vi "New QDList.vi"(8 "error in (no error)":errorcluster, 11 "QDDialogList in":refnum<class "QDDialogList.lvclass">) -> (0 "error out":errorcluster, 3 "QDDialogList out":refnum<class "QDDialogList.lvclass">)   [LabVIEW 2015, in "QDDialogList.lvclass"]
uses:
  QDDialogList.lvclass
  QDDialogList.lvclass/QDDialogList.ctl
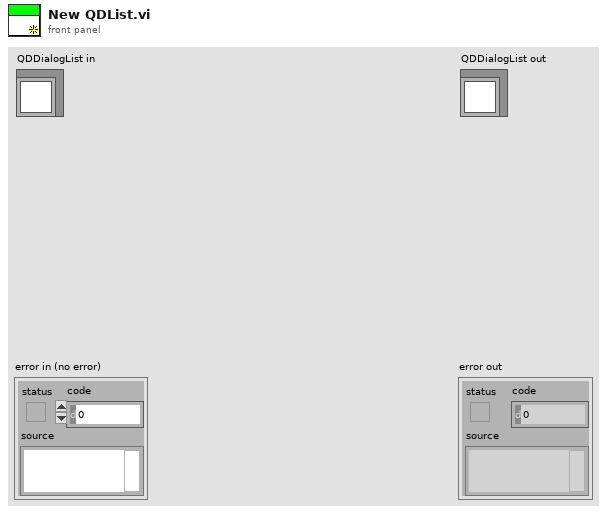
[diagram p1: front panel]
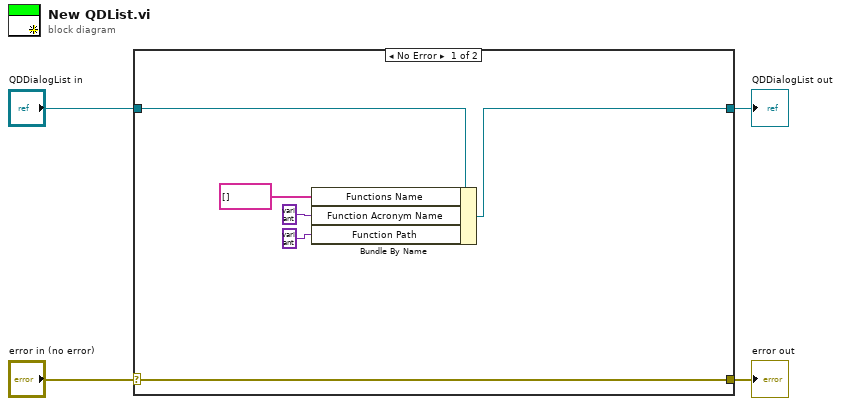
[diagram p0: block diagram]
diagram:
  n1 = case shown="No Error" "error in (no error)" {
    selector: "error in (no error)" -> [w10 w12]
    tunnel: [w10 w12] -> w3
    tunnel: [w5 w11] -> w1
    tunnel: "QDDialogList in" -> [w9 w11]
    frame No Error {
      n2 = Bundle By Name(cluster=w9, "Functions Name"=string[] [], "Function Acronym Name"=variant, "Function Path"=variant) -> (w5:refnum<class "QDDialogList.lvclass">)
    }
    frame Error {
    }
  }
  "error out" <- w3
  "QDDialogList out" <- w1
